vi "Cartesian to Polar.vi"(4 "Cartesian\nCoordinates":cluster{"x":dbl, "y":dbl}) -> (1 "Polar\nCoordinates":cluster{"r":dbl, "theta":dbl})   [LabVIEW 2013]
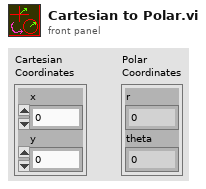
[diagram p1: front panel]
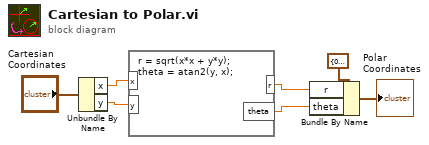
[diagram p0: block diagram]
diagram:
  n1 = Unbundle By Name("Cartesian\nCoordinates") -> ("x"=w4:dbl, "y"=w3:dbl)
  n2 = formula code="r = sqrt(x*x + y*y);\ntheta = atan2(y, x);"("x"=w4, "y"=w3) -> ("r"=w2:dbl, "theta"=w1:dbl)
  n3 = Bundle By Name(cluster=cluster{"r":dbl, "theta":dbl} {"r"=0.0, "theta"=0.0} ("input cluster"), "r"=w2, "theta"=w1) -> (→"Polar\nCoordinates":cluster{"r":dbl, "theta":dbl})
